vi "Clear Strings.vi"(8 "error in (no error)":errorcluster, 11 "BCNavigator in":refnum<class "BreadcrumbNavigator.lvclass">) -> (0 "error out":errorcluster, 3 "BCNavigator out":refnum<class "BreadcrumbNavigator.lvclass">)   [LabVIEW 2015, in "BreadcrumbNavigator.lvclass"]
uses:
  BreadcrumbNavigator.lvclass
  Write Strings[].vi
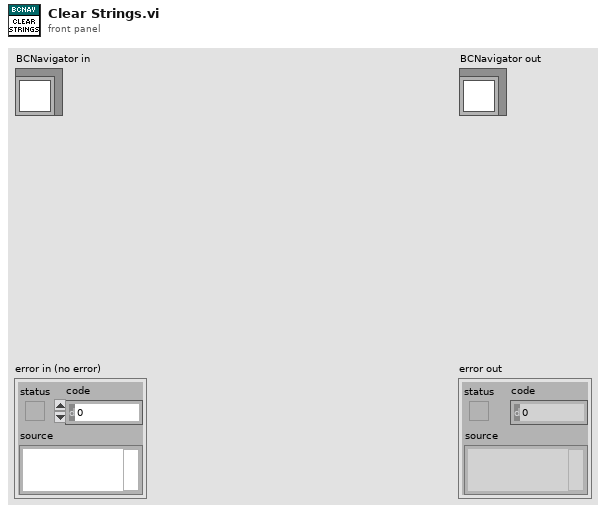
[diagram p1: front panel]
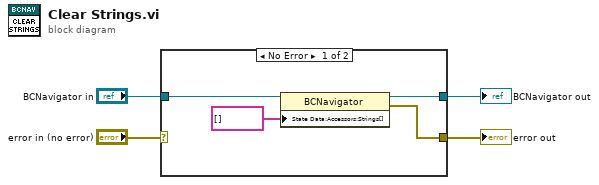
[diagram p0: block diagram]
diagram:
  n1 = case shown="No Error" "error in (no error)" {
    selector: "error in (no error)" -> [_ w10]
    tunnel: [w5 w10] -> w3
    tunnel: [w7 w9] -> w1
    tunnel: "BCNavigator in" -> [w8 w9]
    frame No Error {
      n2 = property class="BCNavigator"(reference=w8, "State Data:Accessors:Strings[]"=string[] [] ("Strings[]")) -> (reference out=w7:refnum<class "BreadcrumbNavigator.lvclass">, error out=w5:errorcluster)  [unwired: 1 in]
    }
    frame Error {
    }
  }
  "error out" <- w3
  "BCNavigator out" <- w1
